vi "LVDimInterface.dim_get_occurrence_ref.vi"(5 "error in (no error)":errorcluster) -> (17 "occurrence":refnum<k4>, 19 "error out":errorcluster)   [LabVIEW 2012, in "LVDimInterface.lvlib"]
doc: "This routine can be called by a server or a client program before to obtain the reference of an occurrence to be fired by the dimWrapper shared library.\n\n\n\nHistory: 24-OCT-2007, Dietrich Beck\n\nCopyright (C)\nGesellschaft für Schwerionenforschung, GSI\nPlanckstr. 1\n64291 Darmstadt\nGermany\n\nContact: D.Beck@gsi.de \n\nThis program is free software; you can redistribute it and/or modify it under the terms of the \nGNU General Public License as published by the Free Software Foundation; either version 2 of the license, or (at your option) any later version.\n\nThis program is distributed in the hope that it will be useful, but WITHOUT ANY WARRANTY; without even the implied warranty of MERCHANTABILITY or FITNESS FOR A PARTICULAR PURPOSE. See the GNU General License for more details (http://www.gnu.org).\n\nGesellschaft für Schwerionenforschung, GSI\nPlanckstr. 1, 64291 Darmstadt, Germany\nFor all questions and ideas contact D. Beck.\nLast update: 16-DEC-2005"
uses:
  LVDimInterface.lvlib
  bin/libDimWrapper.dll
  bin/libDimWrapper.so
  bin/libDimWrapperSPL.dll
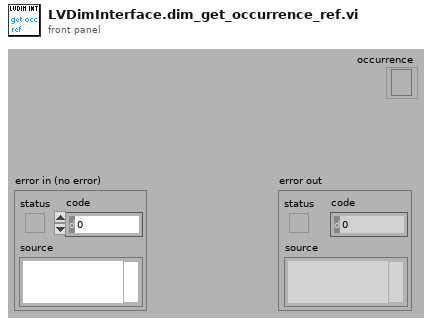
[diagram p1: front panel]
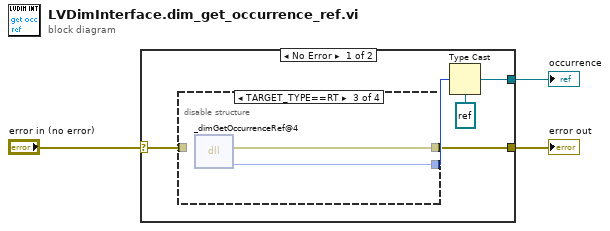
[diagram p0: block diagram]
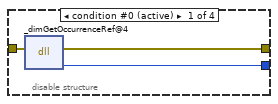
[diagram p2: hidden frame]
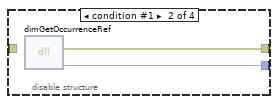
[diagram p3: hidden frame]
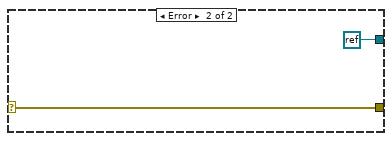
[diagram p5: hidden frame]
diagram:
  n1 = case shown="No Error" "error in (no error)" {
    selector: "error in (no error)" -> [w5 w18]
    tunnel: [w4 w18] -> w3
    tunnel: [w8 refnum<k0> refnum ("Not a Refnum Constant")] -> w1
    frame No Error {
      n2 = disable-structure "Conditional Disable Structure" shown="TARGET_TYPE==RT" {
        disable-tunnel: [w11 w13 w15 _] -> w6
        disable-tunnel: w5 -> [w10 _ _ w16]
        disable-tunnel: [w9 w12 w14 w16] -> w4
        frame condition #0 (active) {
          n3 = dll-call lib="D:/DIMLVEvent LV2012/bin/libDimWrapper.dll" fn="_dimGetOccurrenceRef@4"(error in=w10) -> (error out=w9:errorcluster, "occurrenceRef"=w11:u32)  [unwired: 4 in, 1 out]
        }
        frame condition #1 {
          n4 = dll-call lib="D:/DIMLVEvent LV2012/bin/libDimWrapper.so" fn="dimGetOccurrenceRef" label="libDimWrapper.dll:_dimGetOccurrenceRef@4"() -> (error out=w12:errorcluster, "occurrenceRef"=w13:u32)  [unwired: 5 in, 1 out]
        }
        frame condition #2 {
          n5 = dll-call lib="D:/DIMLVEvent LV2012/bin/libDimWrapperSPL.dll" fn="_dimGetOccurrenceRef@4"() -> (error out=w14:errorcluster, "occurrenceRef"=w15:u32)  [unwired: 5 in, 1 out]
        }
        frame condition #3 {
        }
      }
      n6 = Type Cast(type=refnum<k4> refnum ("occurrence"), x=w6) -> (*(type *) &x=w8:refnum<k4>)
    }
    frame Error {
    }
  }
  "error out" <- w3
  "occurrence" <- w1
